vi "macro_Function_Generator.vi"   [LabVIEW 2019, in "Trajectory_Library.lvlib"]
uses:
  Trajectory_Library.lvlib
  X_Y_PAIR.ctl
types:
  T1 = typedef "Trajectory_Library.lvlib/X_Y_PAIR.ctl" = cluster{"X":dbl, "Y":dbl}
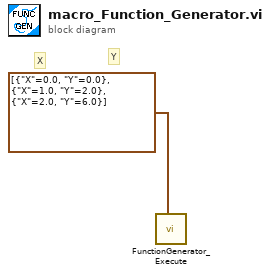
[diagram p0: block diagram]
diagram:
  # "Y"
  # "X"
  n1 = call "FunctionGenerator_Execute.vi"("X Y Pairs"=T1[] [{"X"=0.0, "Y"=0.0}, {"X"=1.0, "Y"=2.0}, {"X"=2.0, "Y"=6.0}]) -> ()  [unwired: 10 in, 1 out]
